vi "loop_demo.vi"() -> ()   [LabVIEW 2014]
panel:
  out "rand":dbl
  out "波形チャート":dbl(graph)
  in  "停止":bool
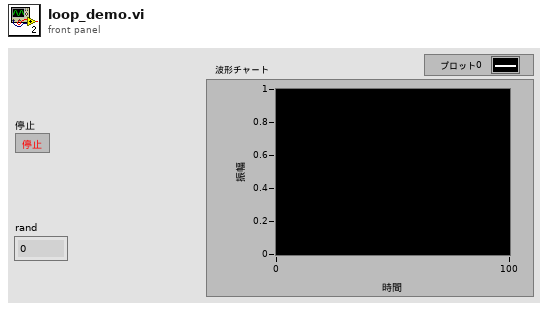
[diagram p1: front panel]
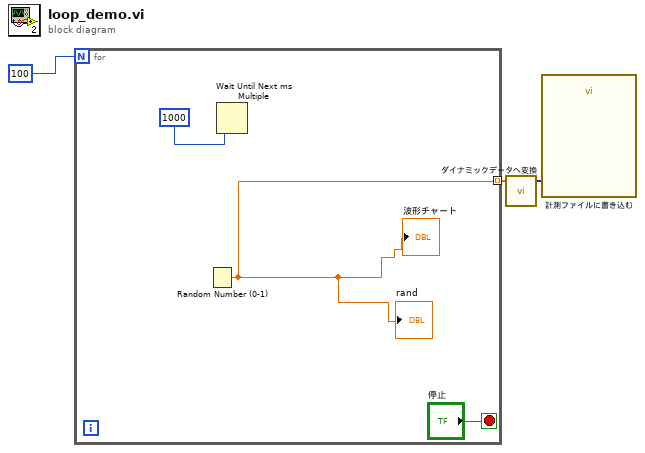
[diagram p0: block diagram]
diagram:
  n1 = for {
    N: 100 -> [_]
    tunnel: [w4] -> w2 mode=indexing
    stop <- "停止" stop-if-true
    n2 = Random Number (0-1)() -> (number: 0 to 1=w4:dbl)
    "波形チャート" <- w4
    "rand" <- w4
    n3 = Wait Until Next ms Multiple(millisecond multiple=1000) -> ()  [unwired: 1 out]
  }
  n4 = call "ダイナミックデータへ変換"("Array"=w2) -> ("Dynamic Data Type"=w1:dynamicdata)  [unwired: 3 in]
  n5 = call "計測ファイルに書き込む"("Signals"=w1) -> ()  [unwired: 16 in, 3 out]
